vi "toml_dump.vi"(4 "vi":refnum<vi>, 8 "error in (no error)":errorcluster, 10 "operation (replace or create)":T1(ring)=enum."replace or create", 11 "path in":path) -> (0 "error out":errorcluster, 2 "file exists":bool, 3 "path out":path)   [LabVIEW 2017]
uses:
  <vilib>/Utility/error.llb/Clear Errors.vi
  toml_lock_obtain.vi
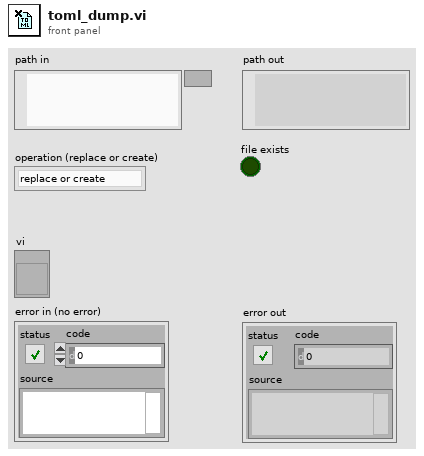
[diagram p1: front panel]
types:
  T1 = enum16{"open", "replace", "create", "open or create", "replace or create", "replace or create with confirmation"}
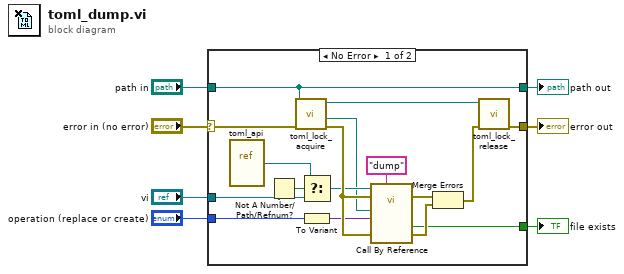
[diagram p0: block diagram]
diagram:
  n1 = case shown="No Error" "error in (no error)" {
    selector: "error in (no error)" -> [w23 w25]
    tunnel: [w19 w25] -> w6
    tunnel: "vi" -> [w16 _]
    tunnel: "path in" -> [w13 w26]
    tunnel: [w13 w26] -> w3
    tunnel: [w11 _] -> w2
    tunnel: "operation (replace or create)" -> [w10 _]
    frame No Error {
      n2 = vi-ref "toml_api.vi"() -> (w15:refnum<vi>)
      n3 = Not A Number/Path/Refnum?(number/path/refnum=w16) -> (NaN/Path/Refnum?=w17:bool)
      n4 = call "toml_lock_acquire.vi"("error in (no error)"=w23, "path in"=w13) -> ("error out"=w22:errorcluster, "resolved path"=w9:path, "lock"=w24:refnum<queue>)  [unwired: 7 in]
      n5 = Select(t=w15, s=w17, f=w16) -> (s? t:f=w14:refnum<vi>)
      n6 = To Variant(anything=w10) -> (Variant=w8:variant)
      n7 = call-by-ref "?"(reference=w14, error in=w22, "cmd"="dump", 8:"error in (no error)"=w22, "data in"=w8, "path in"=w9) -> (error out=w21:errorcluster, 0:"error out"=w12:errorcluster, "return"=w11:bool)  [unwired: 4 in, 3 out]
      n8 = Merge Errors(w21, w12) -> (w20:errorcluster)
      n9 = call "toml_lock_release.vi"("error in (no error)"=w20, "lock"=w24) -> ("error out"=w19:errorcluster)  [unwired: 9 in]
    }
    frame Error {
    }
  }
  "error out" <- w6
  "path out" <- w3
  "file exists" <- w2
